vi "Stop Work.vi"(8 "error in (no error)":errorcluster, 9 "Reply":bool=TRUE, 10 "Reply to":refnum<class "Stop Response Msg.lvclass">, 11 "Measure Object in":refnum<class "Pulse Recorder.lvclass">) -> (0 "error out":errorcluster, 3 "Measure Object out":refnum<class "Pulse Recorder.lvclass">)   [LabVIEW 2016, in "Pulse Recorder.lvclass"]
uses:
  Pulse Recorder.lvclass
  C:/github/LabActor/Template Module/Template Module.lvclass
  Controllers/Process Controller Messages/Stop Response Msg/Stop Response Msg.lvclass
  Pulse Recorder.lvclass/Pulse Recorder.ctl
  Template Module/Template Module.lvclass/Template Module.ctl
  Template Module Messages/Self-Addressed Msg/Self-addressed Msg.lvclass/Self-addressed Msg.ctl
  Controllers/Pulse Controller Messages/Armed Response Msg/Armed Response Msg.lvclass/Armed Response Msg.ctl
  <vilib>/ActorFramework/Message Enqueuer/Message Enqueuer.lvclass/Message Enqueuer.ctl
  Template Module/Read Name.vi
  Template Module/Read Reply to.vi
  Template Module Messages/Self-Addressed Msg/Read Return Enqueuer.vi
  <vilib>/ActorFramework/Message Enqueuer/Enqueue.vi
  Template Module Messages/Result Reply Msg/Result Reply Msg.lvclass
  C:/github/LabActor/Template Module Messages/Self-Addressed Msg/Self-addressed Msg.lvclass
  Controllers/Pulse Controller Messages/Armed Response Msg/Armed Response Msg.lvclass
  C:/Program Files (x86)/National Instruments/LabVIEW 2016/vi.lib/ActorFramework/Message/Message.lvclass
  <vilib>/ActorFramework/Message Priority Queue/Priority Enqueue.vi
  Instrument Actor/Instrument Actor.lvclass
  <vilib>/ActorFramework/Message Enqueuer/Message Enqueuer.lvclass
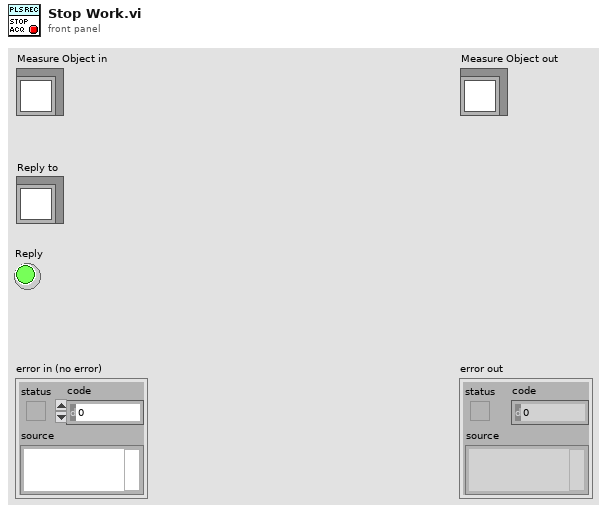
[diagram p1: front panel]
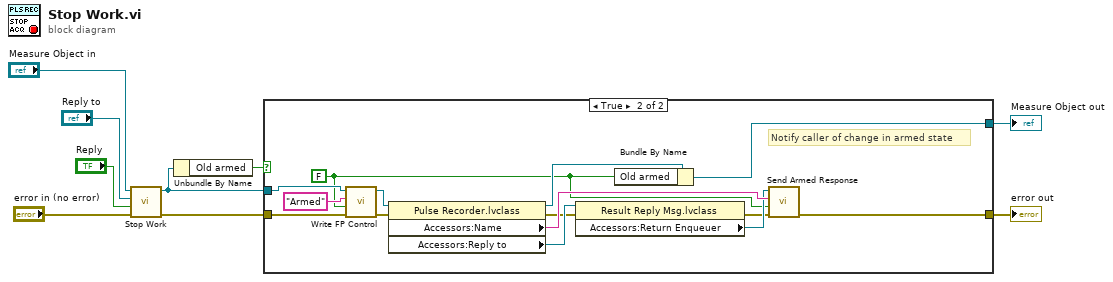
[diagram p0: block diagram]
diagram:
  n1 = call-parent "Stop Work.vi"("error in (no error)"="error in (no error)", "Reply"="Reply", "Reply to"="Reply to", "Measure Object in"="Measure Object in") -> ("error out"=w4:errorcluster, "Measure Object out"=w3:refnum<class "Pulse Recorder.lvclass">)  [unwired: 6 in]
  n2 = Unbundle By Name(w3) -> ("Old armed"=w5:bool)
  n3 = case shown="True" w5 {
    tunnel: w3 -> [w10 w16]
    tunnel: w4 -> [w11 w18]
    tunnel: [w11 w24] -> w1
    tunnel: [w10 w13] -> w2
    frame False {
    }
    frame True {
      w12 = FALSE
      # "Notify caller of change in armed state"
      n4 = call-dynamic "Write FP Control.vi"("error in (no error)"=w18, "Control Value"=w12, "Control Name"="Armed", "Measure Object in"=w16) -> ("error out"=w17:errorcluster, "Measure Object out"=w15:refnum<class "Pulse Recorder.lvclass">)  [unwired: 6 in]
      n5 = property class="Pulse Recorder.lvclass"(reference=w15, error in=w17) -> (reference out=w23:refnum<class "Pulse Recorder.lvclass">, error out=w19:errorcluster, "Accessors:Name"=w25:string, "Accessors:Reply to"=w22:refnum<class "Result Reply Msg.lvclass">)
      n6 = property class="Result Reply Msg.lvclass"(reference=w22, error in=w19) -> (error out=w20:errorcluster, "Accessors:Return Enqueuer"=w21:refnum<class "Message Enqueuer.lvclass">)  [unwired: 1 out]
      n7 = Bundle By Name(cluster=w23, "Old armed"=w12) -> (w13:refnum<class "Pulse Recorder.lvclass">)
      n8 = call "Send Armed Response.vi"("error in (no error)"=w20, "Armed"=w12, "Sender"=w25, "Message Enqueuer"=w21) -> ("error out"=w24:errorcluster)  [unwired: 6 in, 1 out]
    }
  }
  "error out" <- w1
  "Measure Object out" <- w2
